vi "close.vi"(8 "error in (no error)":errorcluster, 11 "PsTti in":refnum<class "PsuTti.lvclass">) -> (0 "error out":errorcluster)   [LabVIEW 2023, in "PsuTti.lvclass"]
doc: "Close the Instrument Reference"
uses:
  PsuTti.lvclass
  PsuTti.lvclass/PsuTti.ctl
  driver/Tti-Pl303Qmd.lvlib
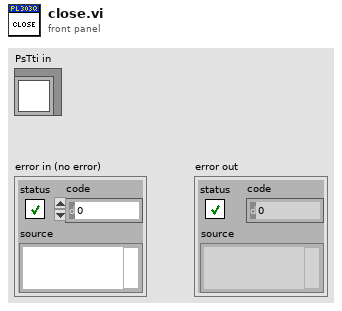
[diagram p1: front panel]
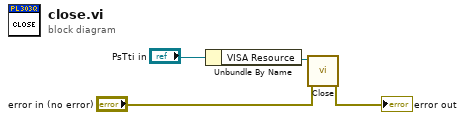
[diagram p0: block diagram]
diagram:
  n1 = Unbundle By Name("PsTti in") -> ("VISA Resource"=w3:refnum<visa-resource-name>)
  n2 = call "Close.vi"("error in (no error)"="error in (no error)", "VISA resource name"=w3) -> ("error out"=→"error out":errorcluster)  [unwired: 9 in]
